vi "GetMatlabArrayInfo.vi"(11 "Value":variant) -> (3 "Array":u32[](array[numeric]))   [LabVIEW 2017]
uses:
  <vilib>/Utility/Data Type/NI_Data Type.lvlib
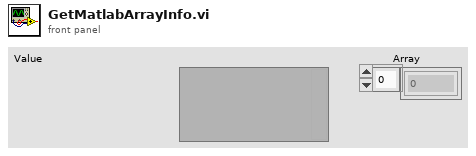
[diagram p1: front panel]
types:
  T1 = typedef "NI_Data Type.lvlib/Memory Info.ctl" = cluster{"Type":T2, "Size":u32}
  T2 = typedef "NI_Data Type.lvlib/Memory Type.ctl" = enum16{"Variable", "Fixed", "Bounded"}
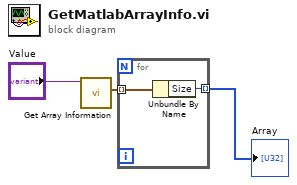
[diagram p0: block diagram]
diagram:
  n1 = call <vilib>:"Get Array Information.vi"("Variant"="Value") -> ("Array Lengths"=w2:T1[])  [unwired: 7 in, 3 out]
  n2 = for {
    tunnel: w2 -> [w5] mode=indexing
    tunnel: [w4] -> w3 mode=indexing
    n3 = Unbundle By Name(w5) -> ("Size"=w4:u32)
  }
  "Array" <- w3
